vi "WriteIntegerGlobals.vi"(0 "controller in":refnum<k24>, 7 "variable number":i32, 9 "values":i32[](array[numeric]), 11 "error in (no error)":errorcluster) -> (4 "controller out":refnum<k24>, 15 "error out":errorcluster)   [LabVIEW 2010]
uses:
  c:/aerotech/controller/5.xx.xxx/ensemble/pc/labview/2010/bin/Aerotech.Ensemble.dll
  bin/Aerotech.Ensemble.dll
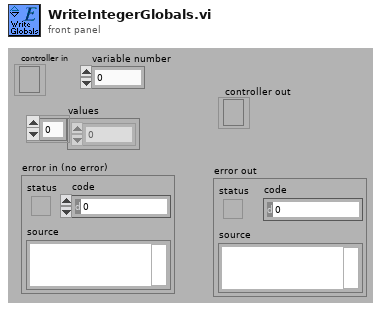
[diagram p1: front panel]
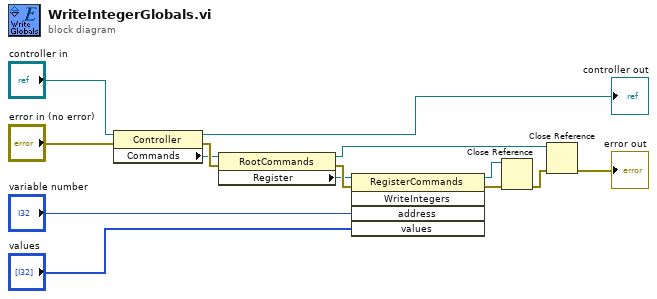
[diagram p0: block diagram]
diagram:
  n1 = property class="Controller"(reference="controller in", error in="error in (no error)") -> (reference out=→"controller out":refnum<k24>, error out=w14:errorcluster, "Commands"=w13:refnum<k24>)
  n2 = property class="RootCommands"(reference=w13, error in=w14) -> (reference out=w8:refnum<k24>, error out=w12:errorcluster, "Register"=w11:refnum<k24>)
  n3 = invoke class="RegisterCommands" method="WriteIntegers"(reference=w11, error in=w12, "address"="variable number", "values"="values") -> (reference out=w10:refnum<k24>, error out=w9:errorcluster)  [unwired: 1 in, 3 out]
  n4 = Close Reference(reference=w10, error in (no error)=w9) -> (error out=w7:errorcluster)
  n5 = Close Reference(reference=w8, error in (no error)=w7) -> (error out=→"error out":errorcluster)
